vi "ConvString.vi"(11 "read buffer":string) -> (3 "Numeric":dbl)   [LabVIEW 2023]
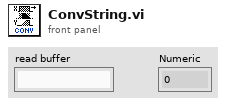
[diagram p1: front panel]
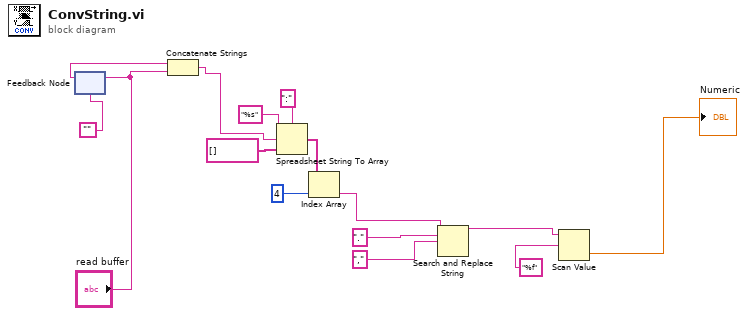
[diagram p0: block diagram]
diagram:
  n1 = feedback #1("") -> (w2:string)
  n2 = feedback-in #1("read buffer") -> ()
  n3 = Concatenate Strings(w2, "read buffer") -> (w15:string)
  n4 = Spreadsheet String To Array(delimiter (Tab)=":", format string="%s", spreadsheet string=w15, array type (2D Dbl)=string[] []) -> (array=w12:string[])
  n5 = Index Array(array=w12, index=4) -> (element=w14:string)
  n6 = Search and Replace String(input string=w14, search string=".", replace string="," ("replace string (\"\")")) -> (result string=w6:string)  [unwired: 5 in, 3 out]
  n7 = Scan Value(string=w6, format string="%f") -> (value=→"Numeric":dbl)  [unwired: 1 in, 1 out]
